vi "AlliGator Single Plot Average Phasor Ratio.vi"(7 "Current Phasor Ref":refnum<vi>, 8 "Error In":errorcluster, 9 "Data":variant, 11 "Registered Events Ctrl Refnums":T1) -> (0 "Error Out":errorcluster, 1 "Message":string)   [LabVIEW 2021, in "AlliGator Phasor Ratio.lvlib"]
doc: "Computes single phasor plot's average phasor ratio."
uses:
  AlliGator Phasor Ratio.lvlib
  GUI/AlliGator Registered Events Ctrl Refnums.ctl
  <vilib>/Utility/miscctls.llb/LVPoint32TypeDef.ctl
  Settings/AlliGator Settings List.ctl
  Phasor/Phasor Ratio Type.ctl
  Phasor/Phasor.lvlib
  Phasor Graph/AlliGator Phasor Graph.lvlib
  Settings/AlliGator Settings.lvlib
  GUI/AlliGator GUI.lvlib
panel:
  # "see the AlliGator License on the block diagram (Ctrl+E or Window:Show Block Diagram)"
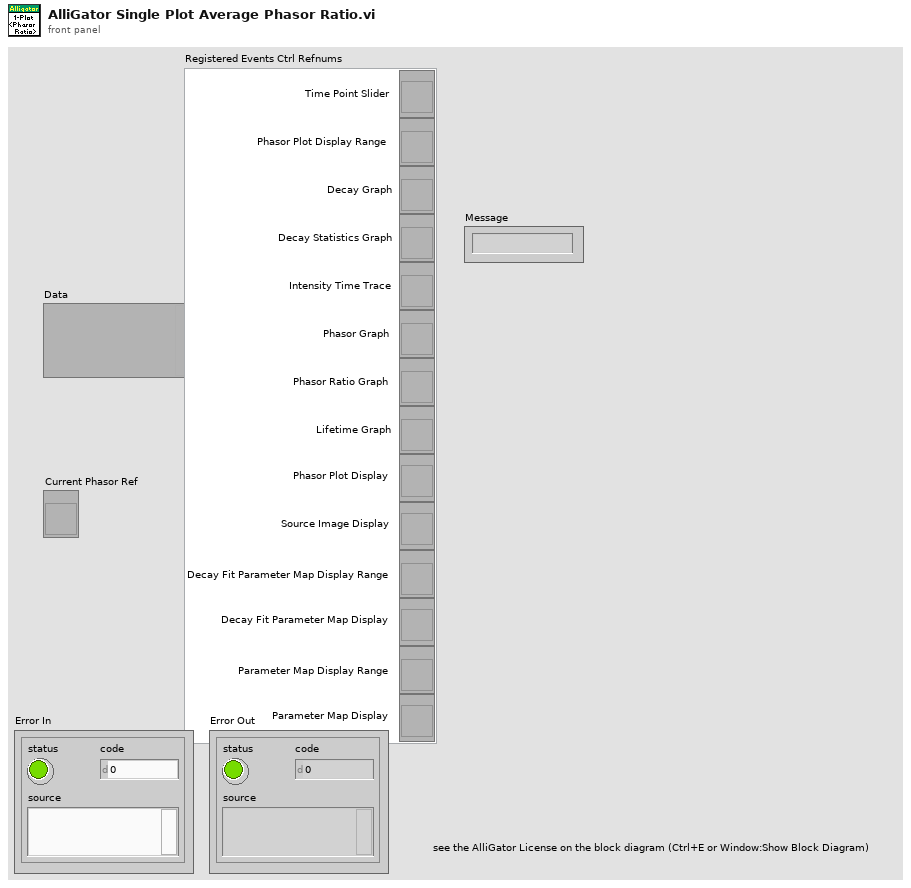
[diagram p1: front panel]
types:
  T1 = typedef "AlliGator GUI.lvlib/AlliGator Registered Events Ctrl Refnums.ctl" = cluster{"Time Point Slider":refnum<vi>, "Phasor Plot Display Range":refnum<vi>, "Decay Graph":refnum<vi>, "Decay Statistics Graph":refnum<vi>, "Intensity Time Trace":refnum<vi>, "Phasor Graph":refnum<vi>, "Phasor Ratio Graph":refnum<vi>, "Lifetime Graph":refnum<vi>, "Phasor Plot Display":refnum<vi>, "Source Image Display":refnum<vi>, "Decay Fit Parameter Map Display Range":refnum<vi>, "Decay Fit Parameter Map Display":refnum<vi>, "Parameter Map Display Range":refnum<vi>, "Parameter Map Display":refnum<vi>}
  T2 = typedef "Phasor.lvlib/Phasor Ratio Type.ctl" = enum32{"Intensity-weighted", "Amplitude-weighted"}
  T3 = typedef "AlliGator Settings.lvlib/AlliGator Settings List.ctl" = enum16{"GUI:Visible Settings Tab", "GUI:Last Run Version", "Source Image:Use Image Histogram for Contrast", "Source Image:Low Count Pixels Rejection Options", "Source Image:High Count Pixels Rejection Options", "Source Image:Use Image Brightness", "Source Image:Blend Overlay with Image Background", "Source Image:Use Fixed ROI Diameter", "Source Image:ROI Diameter", "Source Image:ROI Center Color", "Source Image:Peak Threshold", "Source Image:Intensity Threshold", "Source Image:Image Binning Options", "Source Image:Image Smoothing Options", "Source Image:Image Histogram Active", "Source Image:Invert Binary Mask", "Source Image:Hot Pixel Removal", "Source Image:Overlay Analyzed ROI Center", "Source Image:Auto-Adjust Contrast", "Source Image:Histogram Lower Percentile", "Source Image:Histogram Upper Percentile", "Source Image:Save Source Image", "Source Image:Scale Bar Options", "Source Image:Image Resolution (Pixel Size)", "Source Image:Flatfield Correction", "Source Image:Show Dead Left Columns Correction", "Source Image:Dead Left Columns Correction", "Source Image:Image Pre-Processing Operations Order", "Source Image:Overlay ROI Median", "Source Image:Median Overlay Color", "Data Information:Gate Width", "Data Information:Nanotime Gate Separation", "Data Information:Macrotime Gate Separation", "Data Information:Gate Step", "Data Information:# Gates", "Data Information:Gate Image Exposure", "Data Information:Gate Image Integration", "Data Information:Gates to Skip", "Data Information:Gates to Keep", "Data Information:Define Gates to", "Data Information:Channel Name", "Data Information:Available Channel Names", "Data Information:Channel Arithmetic", "Data Information:Background File Subtraction", "Data Information:Background File", "Data Information:Background Scaling Factor", "Data Information:Background Pile-up Correction", "Data Information:Background Pixel Well Capacity", "Data Information:Laser Period", "Data Information:SYNC Period", "Data Information:Pile-up Correction", "Data Information:Pixel Well Capacity", "Data Information:Dataset Scaling Factor", "Fluorescence Decay_Decay Pre-Processing:Reverse Gates", "Fluorescence Decay_Decay Pre-Processing:Verbose Decay Pre-Processing", "Fluorescence Decay_Decay Pre-Processing:Use Decay Pre-Processing", "Fluorescence Decay_Decay Pre-Processing:Background Subtraction", "Fluorescence Decay_Decay Pre-Processing:Background Definition Range", "Fluorescence Decay_Decay Pre-Processing:Baseline Subtraction Method", "Fluorescence Decay_Decay Pre-Processing:Decay Pre-Processing Operations Order", "Fluorescence Decay_Decay Pre-Processing:Smoothing Parameter", "Fluorescence Decay_Decay Pre-Processing:Shift Decay", "Fluorescence Decay_Decay Pre-Processing:Decay Shift Parameters", "Fluorescence Decay_Decay Pre-Processing:Fold Decay", "Fluorescence Decay_Decay Pre-Processing:# Folds", "Fluorescence Decay_Decay Pre-Processing:1-Normalize Decay", "Fluorescence Decay_Decay Pre-Processing:[0-1]-Normalize Decay", "Fluorescence Decay_Decay Pre-Processing:Smoothen Decay", "Fluorescence Decay_Decay Pre-Processing:Extrapolate Decay", "Fluorescence Decay_Decay Pre-Processing:Use Periodicity", "Fluorescence Decay_Decay Pre-Processing:Use Cursors", "Fluorescence Decay_Decay Pre-Processing:Tail Fraction", "Fluorescence Decay_Decay Pre-Processing:Head Fraction", "Fluorescence Decay_Decay Pre-Processing:Additional Points", "Fluorescence Decay_Decay Pre-Processing:Straighten Decay", "Fluorescence Decay_Decay Pre-Processing:Constant Background", "Fluorescence Decay_Decay Pre-Processing:Pixel-Normalize Decay", "Fluorescence Decay_Advanced Analysis:Extract IRF instead of Decay", "Fluorescence Decay_Advanced Analysis:IRF Extraction Options", "Fluorescence Decay_Advanced Analysis:IRF Optimization Options", "Fluorescence Decay_Advanced Analysis:Square Pulse Options", "Fluorescence Decay_Advanced Analysis:IRF Order", "Fluorescence Decay_Advanced Analysis:IRF Time Constants", "Fluorescence Decay_Advanced Analysis:Wavelet Analysis Options", "Fluorescence Decay_Advanced Analysis:Average Lifetime Options", "Fluorescence Decay_Fit Options:Fit Options", "Fluorescence Decay_Fit Options:Use Legacy Fitting Approach", "Fluorescence Decay_Fit Options:Use Data Information Laser Period", "Fluorescence Decay_Fit Parameters:Displayed Fit Parameters", "Fluorescence Decay_Fit Parameters:Fit Parameter Constraints", "Fluorescence Decay_Fit Parameters:Export Tabulated Results", "Fluorescence Decay_Fit Parameters:MLE Baseline Offset Type", "Fluorescence Decay_Fit Parameters:MLE Baseline Offset", "Fluorescence Decay_Fit Parameters:Guess Parameter Names", "Fluorescence Decay_Fit Parameters:Guess Parameter Values", "Fluorescence Decay_Fit Parameters:Guess Parameters Options", "Fluorescence Decay_Styles:Show Last Decay Only", "Fluorescence Decay_Styles:Decay Graph Color Array", "Fluorescence Decay:Decay Graph Active", "Fluorescence Decay Statistics:Min Peak Value", "Fluorescence Decay Statistics:Reject Low Decay Peak Pixels", "Fluorescence Decay Statistics:Reject High Decay Peak Pixels", "Fluorescence Decay Statistics:Max Peak Value", "Time Traces:Use File Timestamp", "Time Traces:Time Step", "Time Traces:Use Intensity Correction File", "Time Traces:Intensity Correction File", "Phasor Plot:Phasor Plot Smoothing Options", "Phasor Plot:Phasor Plot Size", "Phasor Plot:Phasor Plot Graphics Options", "Phasor Plot:Cumulative Phasor Plot", "Phasor Plot:Use Phasor Brightness", "Phasor Plot:Blend Overlay with Phasor Background", "Phasor Plot:Save Phasor Plot", "Phasor Plot:Show References", "Phasor Plot:Phasor Ratio Decay Range", "Phasor Plot:Exponential Fading", "Phasor Plot:Phasor Ratio Reference Colors", "Phasor Plot:Reference Radius", "Phasor Plot:Show Color Map Vertices", "Phasor Plot:Phasor Plot Active", "Phasor Plot:Phasor Ratio Color Map Type", "Phasor Plot:Phasor Ratio Color Map", "Phasor Plot:Phasor Ratio Display Range", "Phasor Plot:Selected Image ROI(s)", "Phasor Plot:All Image ROIs", "Phasor Plot:Selected Phasor Plot ROI(s)", "Phasor Plot:All Phasor Plot ROIs", "Phasor Plot:Phasor Ratio Color-Coded Quantity", "Phasor Plot:Store Phasor Harmonics", "Phasor Plot:Draw Reference Segment", "Phasor Plot:User-Defined Quantity", "Phasor Graph:Phasor Frequency", "Phasor Graph:Phasor Ratio Type", "Phasor Graph:Pixel-level Phasor Computation", "Phasor Graph:Save Phasor Graph", "Phasor Graph:Phasor Graph Active", "Phasor Graph:Phasor SDV Options", "Phasor Calibration:Use Backup Calibration if needed", "Phasor Graph:Define Shortest Lifetime as", "Phasor Calibration:Backup Calibration Type", "Phasor Calibration:Calibration Type", "Phasor Calibration:Calibration Lifetime", "Phasor Calibration:Calibration Map Algorithm", "Single-Exponential Phasor Locus (SEPL):Gate Parameters", "Single-Exponential Phasor Locus (SEPL):User-defined Gate", "Single-Exponential Phasor Locus (SEPL):User-defined IRF", "Single-Exponential Phasor Locus (SEPL):Phasor Parameters", "Single-Exponential Phasor Locus (SEPL):Decay & IRF Parameters", "Single-Exponential Phasor Locus (SEPL):Display Parameters", "Lifetime Analysis:Decay Analysis Parameters", "Lifetime Analysis:Lifetime Map Active", "Plugins:Python Settings", "Miscellaneous:Verbose Mode", "Miscellaneous:Beep after Script", "Miscellaneous:Saved Image File Format", "Miscellaneous:Exported Gate Image Settings", "Miscellaneous:Include Loading in Timing", "Miscellaneous:Verbose Settings Mode", "Miscellaneous:Histogram Options", "Miscellaneous:Beep on Error", "Miscellaneous:# Logical Processors Used", "Miscellaneous:ROI Description Max Characters", "Miscellaneous:Verbose Error Mode", "Miscellaneous:Transparent Mask Color"}
  T4 = typedef "LVPoint32TypeDef.ctl" = cluster{"Horizontal":i32, "Vertical":i32}
  T5 = typedef "Phasor.lvlib/Phasor (g, s).ctl" = cluster{"g":dbl, "s":dbl}
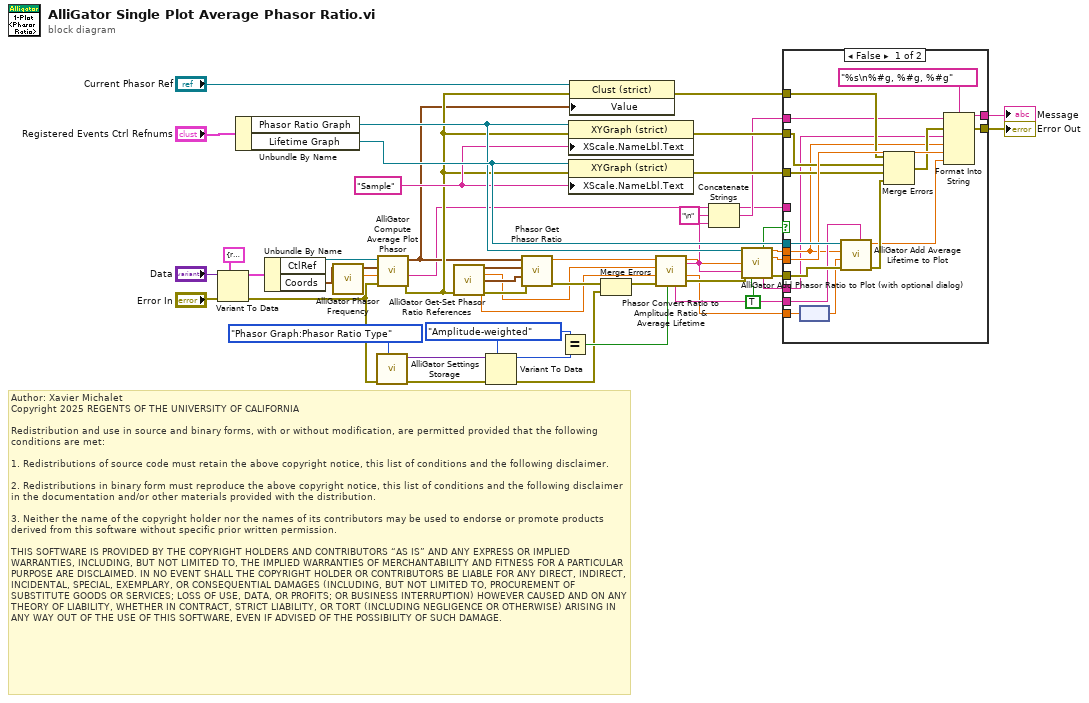
[diagram p0: block diagram]
diagram:
  w7 = Phasor_Ratio_Type."Amplitude-weighted" ("Phasor Ratio Type")
  w39 = "Sample" ("X Scale.Name Label.Text")
  # "Author: Xavier Michalet\nCopyright 2025 REGENTS OF THE UNIVERSITY OF CALIFORNIA\n\nRedistribution and use in source and binary forms, with or without modification, are permitted provided that the following conditions are met:\n\n1. Redistributions of source code must retain the above copyright notice, this list of conditions and the following disclaimer.\n\n2. Redistributions in binary form must reproduce the above copyright notice, this list of conditions and the following disclaimer in the documentation and/or other materials provided with the distribution.\n\n3. Neither the name of the copyright holder nor the names of its contributors may be used to endorse or promote products derived from this software without specific prior written permission.\n\nTHIS SOFTWARE IS PROVIDED BY THE COPYRIGHT HOLDERS AND CONTRIBUTORS “AS IS” AND ANY EXPRESS OR IMPLIED WARRANTIES, INCLUDING, BUT NOT LIMITED TO, THE IMPLIED WARRANTIES OF MERCHANTABILITY AND FITNESS FOR A PARTICULAR PURPOSE ARE DISCLAIMED. IN NO EVENT SHALL THE COPYRIGHT HOLDER OR CONTRIBUTORS BE LIABLE FOR ANY DIRECT, INDIRECT, INCIDENTAL, SPECIAL, EXEMPLARY, OR CONSEQUENTIAL DAMAGES (INCLUDING, BUT NOT LIMITED TO, PROCUREMENT OF SUBSTITUTE GOODS OR SERVICES; LOSS OF USE, DATA, OR PROFITS; OR BUSINESS INTERRUPTION) HOWEVER CAUSED AND ON ANY THEORY OF LIABILITY, WHETHER IN CONTRACT, STRICT LIABILITY, OR TORT (INCLUDING NEGLIGENCE OR OTHERWISE) ARISING IN ANY WAY OUT OF THE USE OF THIS SOFTWARE, EVEN IF ADVISED OF THE POSSIBILITY OF SUCH DAMAGE."
  n1 = Variant To Data(error in="Error In", type=cluster{"CtlRef":refnum<vi>, "Coords":T4} {"CtlRef"=refnum, "Coords"={"Horizontal"=0, "Vertical"=0}} ("output cluster"), Variant="Data") -> (data=w42:cluster{"CtlRef":refnum<vi>, "Coords":T4}, error out=w3:errorcluster)
  n2 = Unbundle By Name("Registered Events Ctrl Refnums") -> ("Phasor Ratio Graph"=w45:refnum<vi>, "Lifetime Graph"=w46:refnum<vi>)
  n3 = Unbundle By Name(w42) -> ("CtlRef"=w26:refnum<vi>, "Coords"=w25:T4)
  n4 = call "AlliGator Phasor Frequency.vi"() -> ("Phasor Frequency"=w23:dbl[unit])
  n5 = call "AlliGator Settings Storage.vi"("AlliGator Settings List"=AlliGator_Settings_List."Phasor Graph:Phasor Ratio Type", "Error In"=w3) -> ("Error Out"=w8:errorcluster, "Variant Data out"=w9:variant)  [unwired: 8 in]
  n6 = call "AlliGator Compute Average Plot Phasor.vi"("error in (no error)"=w3, "Phasor Frequency"=w23, "Mouse Click Coordinates"=w25, "XYGraph Ref"=w26) -> ("error out"=w24:errorcluster, "Result String"=w15:string, "Phasor (g, s)"=w19:T5)  [unwired: 4 in, 1 out]
  n7 = call "AlliGator Get-Set Phasor Ratio References.vi"("error in (no error)"=w24) -> ("Reference Phasor 1"=w33:T5, "Reference Lifetime 1"=w17:dbl[unit], "Reference Phasor 2"=w32:T5, "Reference Lifetime 2"=w16:dbl[unit], "error out"=w31:errorcluster)  [unwired: 7 in, 3 out]
  n8 = Variant To Data(error in=w8, type=w7, Variant=w9) -> (data=w10:T2, error out=w1:errorcluster)
  n9 = call "Phasor Get Phasor Ratio.vi"("Error In"=w31, "Reference Phasor 2"=w32, "Reference Phasor 1"=w33, "Phasor"=w19) -> ("Error Out"=w41:errorcluster, "Phasor Ratio (f1)"=w40:dbl)  [unwired: 5 in, 1 out]
  n10 = Equal?(x=w7, y=w10) -> (x = y?=w6:bool)
  n11 = property class="XYGraph (strict)"(reference=w45, error in=w24, "XScale.NameLbl.Text"=w39) -> (error out=w29:errorcluster)  [unwired: 1 out]
  n12 = property class="XYGraph (strict)"(reference=w46, error in=w24, "XScale.NameLbl.Text"=w39) -> (error out=w30:errorcluster)  [unwired: 1 out]
  n13 = property class="Clust (strict)"(reference="Current Phasor Ref", error in=w24, "Value"=w19) -> (error out=w28:errorcluster)  [unwired: 1 out]
  n14 = Merge Errors(w41, w1) -> (w2:errorcluster)
  n15 = call "Phasor Convert Ratio to Amplitude Ratio & Average Lifetime.vi"("Compute Amplitude Ratio"=w6, "error in (no error)"=w2, "Reference Lifetime 2"=w16, "Reference Lifetime 1"=w17, "Phasor Ratio (f1)"=w40) -> ("error out"=w37:errorcluster, "Average Lifetime"=w4:dbl[unit], "Phasor/Amplitude Ratio"=w36:dbl, "Average Lifetime Caption"=w14:string, "Phasor Ratio Plot Name Suffix"=w18:string)  [unwired: 2 in]
  n16 = Concatenate Strings(w15, "\n" ("string"), w18) -> (w22:string)
  n17 = call "AlliGator Add Phasor Ratio to Plot (with optional dialog).vi"("XYGraph in"=w45, "Phasor Ratio"=w36, "error in (no error)"=w37, "Interactive?"=TRUE, "New Plot Name"=w18) -> ("Cancelled?"=w20:bool, "Sample Abscissa"=w35:dbl, "Phasor Ratio"=w34:dbl, "Message"=w5:string, "error out"=w38:errorcluster)  [unwired: 5 in, 1 out]
  n18 = case shown="False" w20 {
    tunnel: w46 -> [w67 _]
    tunnel: [w66 w68] -> w11
    tunnel: [w65 _] -> w12
    tunnel: w38 -> [w64 w68]
    tunnel: w35 -> [w53 _]
    tunnel: w34 -> [w63 _]
    tunnel: w30 -> [w60 _]
    tunnel: w29 -> [w59 _]
    tunnel: w28 -> [w57 _]
    tunnel: w22 -> [w56 _]
    tunnel: w15 -> [_ _]
    tunnel: w14 -> [w54 _]
    tunnel: w5 -> [w52 _]
    tunnel: w4 -> [w51 _]
    frame False {
      n19 = node(w51) -> (w50:dbl)
      n20 = call "AlliGator Add Average Lifetime to Plot.vi"("New Plot Name"=w54, "error in (no error)"=w64, "Average Lifetime"=w50, "Abscissa"=w53, "Lifetime Graph refnum"=w67) -> ("error out"=w62:errorcluster, "Average Lifetime (dup)"=w58:dbl)  [unwired: 3 in, 2 out]
      n21 = Merge Errors(w57, w59, w60, w62) -> (w61:errorcluster)
      n22 = Format Into String(format string="%s\n%#g, %#g, %#g", initial string=w56, error in=w61, w52, w53, w63, w58) -> (resulting string=w65:string, error out=w66:errorcluster)
    }
    frame True {
    }
  }
  "Error Out" <- w11
  "Message" <- w12
